vi "Update Sensor Data.vi"(8 "error in (no error)":errorcluster, 10 "SensorData":refnum<class "SensorData.lvclass">, 11 "SensorView in":refnum<class "SensorView.lvclass">) -> (0 "error out":errorcluster, 3 "SensorView out":refnum<class "SensorView.lvclass">)   [LabVIEW 2012, in "Sensor Definition.lvlib" / "SensorView.lvclass"]
uses:
  SensorView.lvclass
  SensorData.lvclass
  Double Scalar SensorData.lvclass
  SensorView.lvclass/SensorView.ctl
  Read SensorData.vi
  Read SensorData Changed Event.vi
  Write SensorData.vi
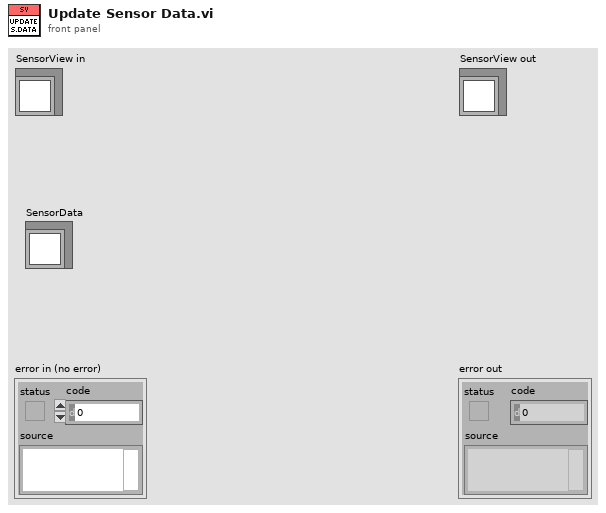
[diagram p1: front panel]
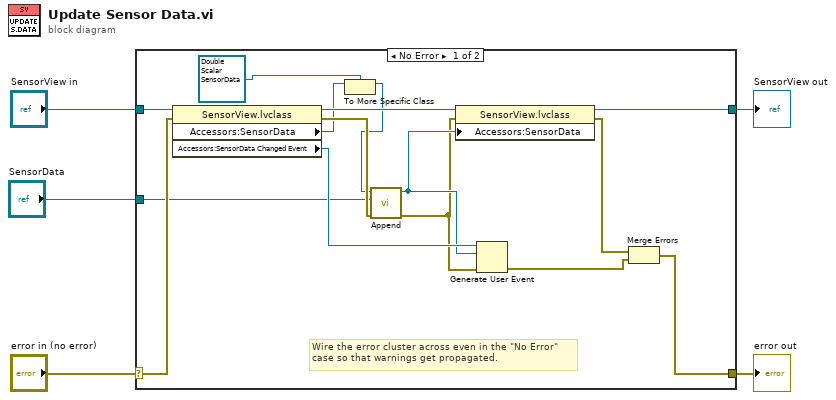
[diagram p0: block diagram]
diagram:
  n1 = case shown="No Error" "error in (no error)" {
    selector: "error in (no error)" -> [w11 w22]
    tunnel: [w10 w22] -> w4
    tunnel: [w18 w21] -> w2
    tunnel: "SensorView in" -> [w20 w21]
    tunnel: "SensorData" -> [w9 _]
    frame No Error {
      # "Wire the error cluster across even in the \"No Error\"\ncase so that warnings get propagated."
      n2 = property class="SensorView.lvclass"(reference=w20, error in=w11) -> (reference out=w19:refnum<class "SensorView.lvclass">, error out=w15:errorcluster, "Accessors:SensorData"=w8:refnum<class "SensorData.lvclass">, "Accessors:SensorData Changed Event"=w17:refnum<user-event>)
      n3 = To More Specific Class(target class=refnum<class "Double Scalar SensorData.lvclass"> refnum ("Sensor Definition.lvlib:Double Scalar SensorData.lvclass"), reference=w8) -> (specific class reference=w7:refnum<class "Double Scalar SensorData.lvclass">)  [unwired: 1 in, 1 out]
      n4 = call-dynamic "Append.vi"("error in (no error)"=w15, "SensorData in 2"=w9, "Double Scalar SensorData in"=w7) -> ("error out"=w14:errorcluster, "Double Scalar SensorData out"=w16:refnum<class "Double Scalar SensorData.lvclass">)  [unwired: 7 in]
      n5 = property class="SensorView.lvclass"(reference=w19, error in=w14, "Accessors:SensorData"=w16) -> (reference out=w18:refnum<class "SensorView.lvclass">, error out=w13:errorcluster)
      n6 = Generate User Event(user event=w17, event data cluster=w16, error in=w14) -> (error out=w12:errorcluster)  [unwired: 1 out]
      n7 = Merge Errors(w13, w12) -> (w10:errorcluster)
    }
    frame Error {
    }
  }
  "error out" <- w4
  "SensorView out" <- w2
